vi "Get All RFmx VNA Sessions with Tester Type.vi"(0 "TSM Context In":T1, 5 "Tester Type":string="RFPM", 11 "error in":errorcluster) -> (4 "TSM Context Out":T1, 6 "RFmx VNA Sessions":refnum<k21>[](array[refnum]), 15 "error out":errorcluster)   [LabVIEW 2023, in "RFCalAndFixtureCharact.Common.lvlib"]
uses:
  <vilib>/NI_TestStand_SemiconductorModule/NI_TestStand_Semiconductor_Module.lvlibp/PinMap/General/SemiconductorModuleContext.ctl
  Global Data Id Prefix.vi
  <vilib>/NI_TestStand_SemiconductorModule/NI_TestStand_Semiconductor_Module.lvlibp/PinMap/Site and Global Data/GlobalDataExists.vi
  <vilib>/NI_TestStand_SemiconductorModule/NI_TestStand_Semiconductor_Module.lvlibp/PinMap/Site and Global Data/GetGlobalData.vi
  <vilib>/Utility/error.llb/Error Cluster From Error Code.vi
  <vilib>/ErrorRing/Error Ring.xnode
  RFCalAndFixtureCharact.Common.lvlib
  <vilib>/NI_TestStand_SemiconductorModule/NI_TestStand_Semiconductor_Module.lvlibp
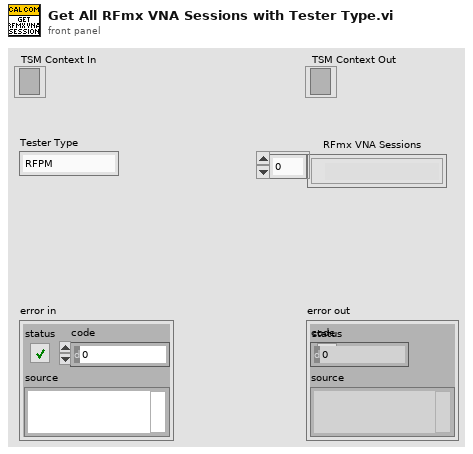
[diagram p1: front panel]
types:
  T1 = typedef "NI_TestStand_Semiconductor_Module.lvlibp/SemiconductorModuleContext.ctl" = refnum<k7>
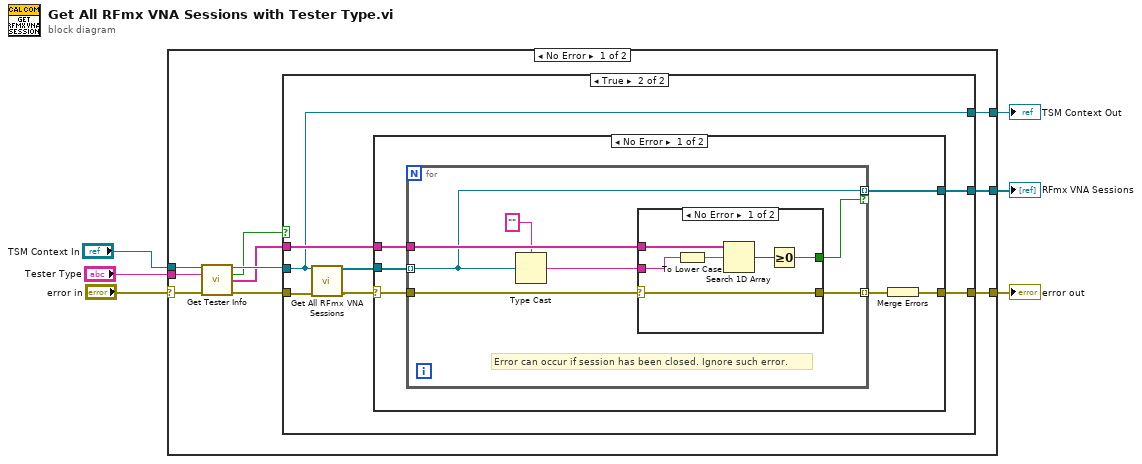
[diagram p0: block diagram]
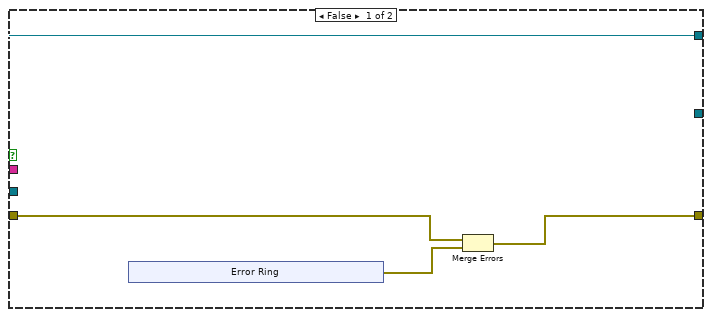
[diagram p2: hidden frame]
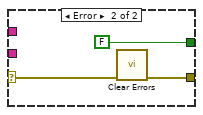
[diagram p3: hidden frame]
diagram:
  n1 = case shown="No Error" "error in" {
    selector: "error in" -> [w9 w56]
    tunnel: "TSM Context In" -> [w16 w57]
    tunnel: [w15 w56] -> w5
    tunnel: [w14 _] -> w1
    tunnel: "Tester Type" -> [w13 _]
    tunnel: [w12 w57] -> w3
    frame No Error {
      n2 = call "Get Tester Info.vi"("TSM Context In"=w16, "Tester Type"=w13, "error in"=w9) -> ("TSM Context Out"=w10:T1, "Resource Descriptors Exist?"=w7:bool, "Resource Descriptors"=w8:string[], "error out"=w11:errorcluster)  [unwired: 8 in, 1 out]
      n3 = case shown="True" w7 {
        tunnel: w8 -> [_ w32]
        tunnel: w11 -> [w18 w28]
        tunnel: [w19 w31] -> w15
        tunnel: [_ w30] -> w14
        tunnel: w10 -> [w17 w29]
        tunnel: [w17 w29] -> w12
        frame False {
          n4 = xnode "Error Ring"() -> ("error out"=w20:errorcluster)
          n5 = Merge Errors(w18, w20) -> (w19:errorcluster)
        }
        frame True {
          n6 = call "Get All RFmx VNA Sessions.vi"("TSM Context"=w29, "error in"=w28) -> ("RFmx VNA Sessions"=w26:refnum<k21>[], "error out"=w27:errorcluster)  [unwired: 12 in]
          n7 = case shown="No Error" w27 {
            selector: w27 -> [w36 w55]
            tunnel: w26 -> [w38 _]
            tunnel: w32 -> [w37 _]
            tunnel: [w34 w55] -> w31
            tunnel: [w33 _] -> w30
            frame No Error {
              n8 = for {
                tunnel: w36 -> [w42]
                tunnel: w38 -> [w41] mode=indexing
                tunnel: w37 -> [w45]
                tunnel: [w41] -> w33 mode=indexing if=w44
                tunnel: [w43] -> w35 mode=indexing
                # "Error can occur if session has been closed. Ignore such error."
                n9 = Type Cast(type="", x=w41) -> (*(type *) &x=w40:string)
                n10 = case shown="No Error" w42 {
                  selector: w42 -> [w48 w53]
                  tunnel: w45 -> [w51 _]
                  tunnel: [w49 FALSE] -> w44
                  tunnel: [w48 w52] -> w43
                  tunnel: w40 -> [w46 _]
                  frame No Error {
                    n11 = To Lower Case(string=w46) -> (all lower case string=w47:string)
                    n12 = Search 1D Array(1D array=w51, element=w47) -> (index of element=w50:i32)  [unwired: 1 in]
                    n13 = Greater Or Equal To 0?(x=w50) -> (x >= 0?=w49:bool)
                  }
                  frame Error {
                    n14 = call <vilib>:"Clear Errors.vi"("error in (no error)"=w53) -> ("error out"=w52:errorcluster)  [unwired: 5 in, 1 out]
                  }
                }
              }
              n15 = Merge Errors(w35) -> (w34:errorcluster)
            }
            frame Error {
            }
          }
        }
      }
    }
    frame Error {
    }
  }
  "TSM Context Out" <- w3
  "error out" <- w5
  "RFmx VNA Sessions" <- w1
